vi "validate line configuration.vi"(7 "modbus":refnum<class "Modbus Slave configuration.lvclass">, 11 "line in":T1) -> (1 "valid?":bool, 2 "issues":string, 3 "line out":T1)   [LabVIEW 2013, in "Modbus Slave editor node.lvclass"]
doc: "Platypus Framework 1.0.1.65\nNI Systems Engineering - National Instruments"
uses:
  Modbus Slave editor node.lvclass
  table line.ctl
  <vilib>/NI/TBM Modules/modbus slave/module channel/Modbus Module Channel.lvclass
  <vilib>/NI/TBM Modules/modbus slave/configuration/Modbus Slave configuration.lvclass
  <vilib>/NI/Tag Bus/tag/tag descriptor.lvclass/tag descriptor.ctl
  <vilib>/NI/TBM Modules/modbus slave/module channel/Modbus Module Channel.lvclass/Modbus Module Channel.ctl
  <vilib>/NI/Tag Bus/tag/Data Type.ctl
  <vilib>/NI/Tag Bus/tag/read tag name.vi
  <vilib>/NI/Tag Bus/tag/read data type.vi
  <vilib>/NI/TBM Modules/modbus slave/module channel/Read modbus type.vi
  <vilib>/NI/Tag Bus/tag/tag descriptor.lvclass
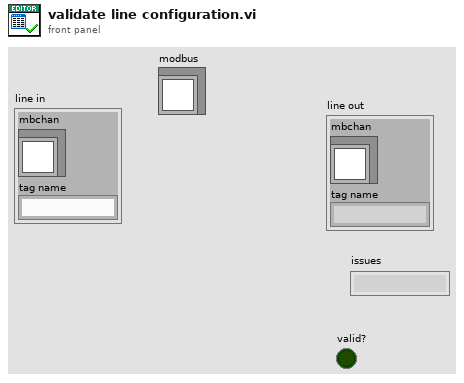
[diagram p1: front panel]
types:
  T1 = typedef "Modbus Slave editor node.lvclass/table line.ctl" = cluster{"mbchan":refnum<class "Modbus Module Channel.lvclass">, "tag name":string}
  T2 = typedef "tag bus.lvlib/tag descriptor.lvclass/Data Type.ctl" = enum16{"Double", "Single", "I64", "I32", "I16", "I8", "U64", "U32", "U16", "U8", "Boolean", "String", "Array of Double", "Array of Single", "Array of I64", "Array of I32", "Array of I16", "Array of I8", "Array of U64", "Array of U32", "Array of U16", "Array of U8", "Array of Boolean", "Array of String"}
  T3 = typedef "Modbus Module Channel.lvclass/data bank type.ctl" = enum16{"coils", "discrete inputs", "input registers", "holding registers"}
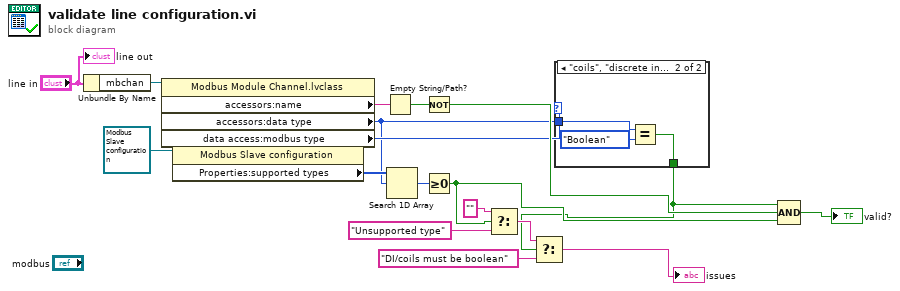
[diagram p0: block diagram]
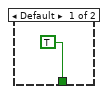
[diagram p2: hidden frame]
diagram:
  n1 = Unbundle By Name("line in") -> ("mbchan"=w17:refnum<class "Modbus Module Channel.lvclass">)
  n2 = property class="Modbus Module Channel.lvclass"(reference=w17) -> ("accessors:name"=w16:string, "accessors:data type"=w5:T2, "data access:modbus type"=w6:T3)  [unwired: 1 in, 2 out]
  n3 = property class="Modbus Slave configuration"(reference=refnum<class "Modbus Slave configuration.lvclass"> refnum ("tag bus configurable plugin module configuration")) -> ("Properties:supported types"=w12:T2[])  [unwired: 1 in, 2 out]
  n4 = Empty String/Path?(string/path=w16) -> (empty?=w15:bool)
  n5 = Search 1D Array(1D array=w12, element=w5) -> (index of element=w10:i32)  [unwired: 1 in]
  n6 = Not(x=w15) -> (.not. x?=w14:bool)
  n7 = Greater Or Equal To 0?(x=w10) -> (x >= 0?=w9:bool)
  n8 = Select(t="", s=w9, f="Unsupported type") -> (s? t:f=w4:string)
  n9 = case shown="\"coils\", \"discrete inputs\"" w6 {
    tunnel: [TRUE w22] -> w2
    tunnel: w5 -> [_ w21]
    frame Default {
    }
    frame "coils", "discrete inputs" {
      n10 = Equal?(x=w21, y=Data_Type."Boolean") -> (x = y?=w22:bool)
    }
  }
  n11 = Select(t=w4, s=w2, f="DI/coils must be boolean") -> (s? t:f=→"issues":string)
  n12 = Compound Arithmetic op=AND(w2, w14, w9) -> (→"valid?":bool)
  "line out" <- "line in"
